vi "SetFrameColor.vi"(8 "error in (no error)":errorcluster, 10 "frame color":u32(colorbox)=9868950, 11 "menu in":refnum<class "menu.lvclass">) -> (0 "error out":errorcluster, 3 "menu out":refnum<class "menu.lvclass">)   [LabVIEW 2009, in "menu.lvclass"]
uses:
  menu.lvclass
  menu.lvclass/menu.ctl
  Frame/frame.lvclass
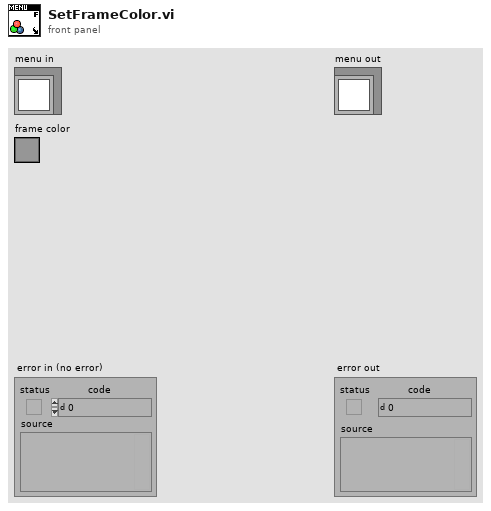
[diagram p1: front panel]
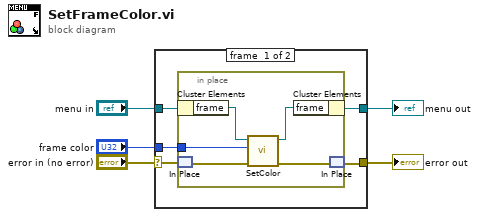
[diagram p0: block diagram]
diagram:
  n1 = case shown="No Error" "error in (no error)" {
    selector: "error in (no error)" -> [w8 w17]
    tunnel: [w7 w17] -> w2
    tunnel: [w9 w16] -> w4
    tunnel: "menu in" -> [w10 w16]
    tunnel: "frame color" -> [w6 _]
    frame #0 {
      n2 = in-place {
        in-place-border: w6 -> [w11]
        n3 = in-place-cluster #1(w10) -> ("frame"=w13:refnum<class "frame.lvclass">)
        n4 = in-place-match #2(w8) -> (w15:errorcluster)
        n5 = call "SetColor.vi"("error in (no error)"=w15, "color"=w11, "frame in"=w13) -> ("error out"=w14:errorcluster, "frame out"=w12:refnum<class "frame.lvclass">)  [unwired: 7 in]
        n6 = in-place-cluster #1("frame"=w12) -> (w9:refnum<class "menu.lvclass">)
        n7 = in-place-match #2(w14) -> (w7:errorcluster)
      }
    }
    frame #1 {
    }
  }
  "menu out" <- w4
  "error out" <- w2
